vi "Read Active Path.vi"(8 "error in (no error)":errorcluster, 11 "Setting Database in":refnum<class "Setting Database.lvclass">) -> (0 "error out":errorcluster, 2 "Path Settings.lvclass":refnum<class "Path Settings.lvclass">, 3 "Setting Database out":refnum<class "Setting Database.lvclass">)   [LabVIEW 2019, in "Setting Database.lvclass"]
uses:
  Setting Database.lvclass
  Path Settings/Path Settings.lvclass
  Setting Database.lvclass/Setting Database.ctl
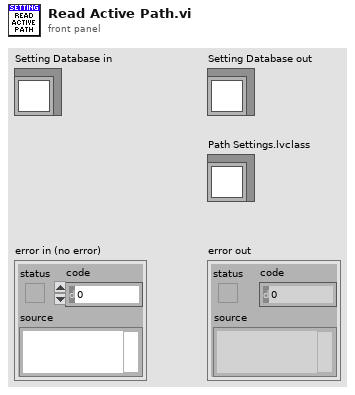
[diagram p1: front panel]
types:
  T1 = cluster{"Path":i32, "Funnel":i32, "Rectangle":i32, "Dot":i32}
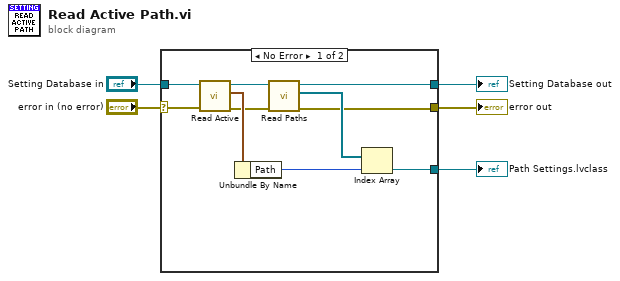
[diagram p0: block diagram]
diagram:
  n1 = case shown="No Error" "error in (no error)" {
    selector: "error in (no error)" -> [w8 w16]
    tunnel: [w6 w16] -> w4
    tunnel: [w14 w17] -> w2
    tunnel: "Setting Database in" -> [w12 w17]
    tunnel: [w15 _] -> w1
    frame No Error {
      n2 = call "Read Active.vi"("error in (no error)"=w8, "Setting Database in"=w12) -> ("error out"=w7:errorcluster, "Active"=w11:T1, "Setting Database out"=w13:refnum<class "Setting Database.lvclass">)  [unwired: 7 in]
      n3 = Unbundle By Name(w11) -> ("Path"=w9:i32)
      n4 = call "Read Paths.vi"("error in (no error)"=w7, "Setting Database in"=w13) -> ("error out"=w6:errorcluster, "Paths"=w10:refnum<class "Path Settings.lvclass">[], "Setting Database out"=w14:refnum<class "Setting Database.lvclass">)  [unwired: 7 in]
      n5 = Index Array(array=w10, index=w9) -> (element=w15:refnum<class "Path Settings.lvclass">)
    }
    frame Error {
    }
  }
  "error out" <- w4
  "Setting Database out" <- w2
  "Path Settings.lvclass" <- w1
